vi "test5.vi"() -> ()   [LabVIEW 2014]
panel:
  in  "Rang N":i32
  out "Tableau":dbl[](array[numeric])
  out "?":dbl[](graph)
  in  "?":bool
  in  "?":bool
  in  "?":bool
  in  "?":bool
  in  "?":bool
  in  "?":bool
  in  "?":bool
  in  "?":bool
  in  "?":bool
  in  "?":bool
  out "Minimum":dbl
  out "Maximum":dbl
  out "Moyenne":dbl
  in  "Valeur":dbl
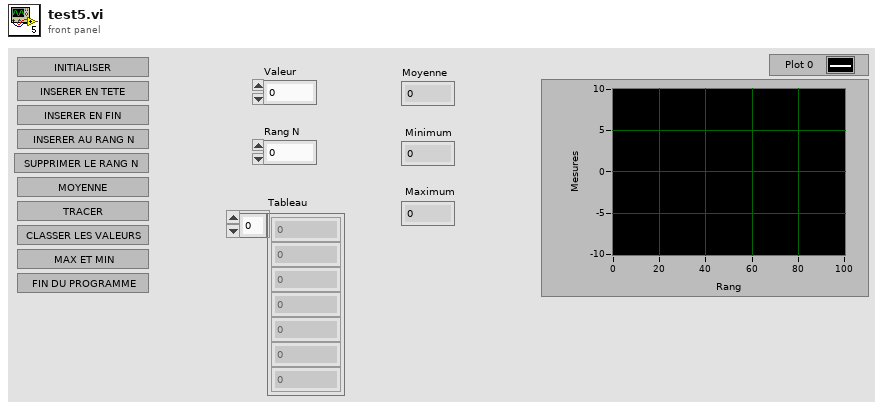
[diagram p1: front panel]
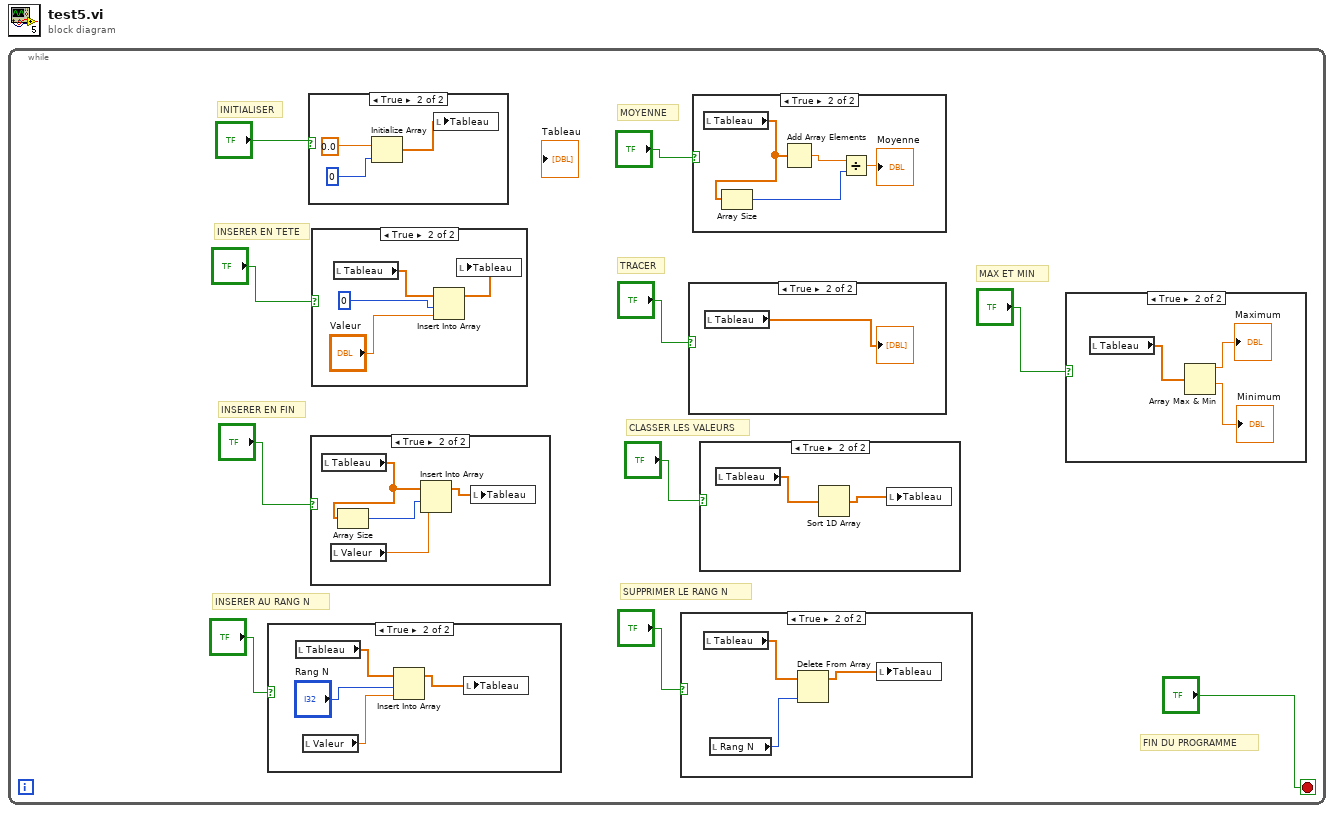
[diagram p0: block diagram]
diagram:
  n1 = while {
    stop <- "?" stop-if-true
    # "FIN DU PROGRAMME"
    # "MAX ET MIN"
    # "CLASSER LES VALEURS"
    # "TRACER"
    # "MOYENNE"
    # "SUPPRIMER LE RANG N"
    # "INSERER AU RANG N"
    # "INSERER EN FIN"
    # "INSERER EN TETE"
    # "INITIALISER"
    n2 = case shown="True" "?" {
      frame False {
      }
      frame True {
        n3 = local read "Tableau"() -> (w21:dbl[])
        n4 = local read "Valeur"() -> (w20:dbl)
        n5 = Insert Into Array(array=w21, index="Rang N", new element=w20) -> (w19:dbl[])
        n6 = local write "Tableau"(w19) -> ()
      }
    }
    n7 = case shown="True" "?" {
      frame False {
      }
      frame True {
        n8 = Initialize Array(0.0, 0) -> (w36:dbl[])
        n9 = local write "Tableau"(w36) -> ()
      }
    }
    n10 = case shown="True" "?" {
      frame False {
      }
      frame True {
        n11 = local read "Tableau"() -> (w25:dbl[])
        n12 = local read "Valeur"() -> (w24:dbl)
        n13 = Array Size(array=w25) -> (size(s)=w26:i32)
        n14 = Insert Into Array(array=w25, index=w26, new element=w24) -> (w23:dbl[])
        n15 = local write "Tableau"(w23) -> ()
      }
    }
    n16 = case shown="True" "?" {
      frame False {
      }
      frame True {
        n17 = local read "Tableau"() -> (w31:dbl[])
        n18 = Insert Into Array(array=w31, index=0, new element="Valeur") -> (w28:dbl[])
        n19 = local write "Tableau"(w28) -> ()
      }
    }
    n20 = case shown="True" "?" {
      frame False {
      }
      frame True {
        n21 = local read "Tableau"() -> (w18:dbl[])
        n22 = local read "Rang N"() -> (w17:i32)
        n23 = Delete From Array(array=w18, index=w17) -> (array with subset deleted=w16:dbl[])  [unwired: 1 in, 1 out]
        n24 = local write "Tableau"(w16) -> ()
      }
    }
    n25 = case shown="True" "?" {
      frame False {
      }
      frame True {
        n26 = local read "Tableau"() -> (→"?":dbl[])
      }
    }
    n27 = case shown="True" "?" {
      frame False {
      }
      frame True {
        n28 = local read "Tableau"() -> (w35:dbl[])
        n29 = Array Size(array=w35) -> (size(s)=w33:i32)
        n30 = Add Array Elements(numeric array=w35) -> (sum=w34:dbl)
        n31 = Divide(x=w34, y=w33) -> (x/y=→"Moyenne":dbl)
      }
    }
    n32 = case shown="True" "?" {
      frame False {
      }
      frame True {
        n33 = local read "Tableau"() -> (w15:dbl[])
        n34 = Sort 1D Array(array=w15) -> (sorted array=w14:dbl[])
        n35 = local write "Tableau"(w14) -> ()
      }
    }
    n36 = case shown="True" "?" {
      frame False {
      }
      frame True {
        n37 = local read "Tableau"() -> (w13:dbl[])
        n38 = Array Max & Min(array=w13) -> (max value=→"Maximum":dbl, min value=→"Minimum":dbl)  [unwired: 2 out]
      }
    }
  }
